vi "Auto_Routine_StraightTwoPiece.vi"(8 "error in (no error)":errorcluster) -> (0 "error out":errorcluster)   [LabVIEW 2023]
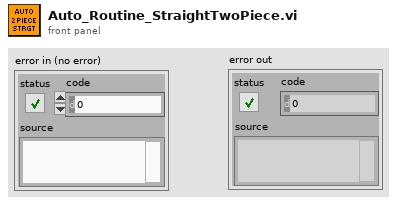
[diagram p1: front panel]
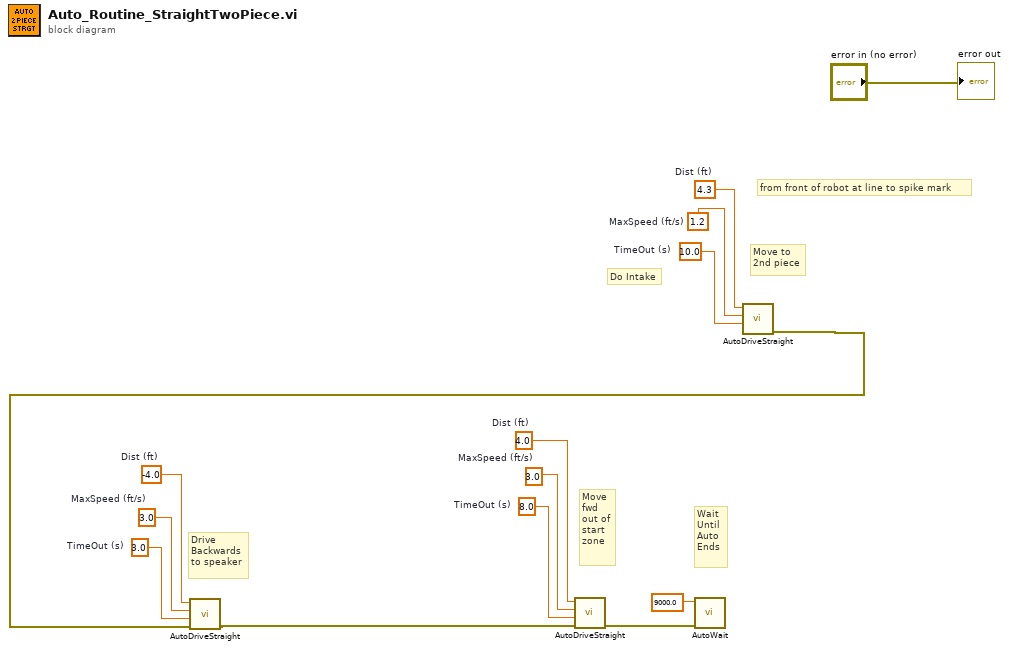
[diagram p0: block diagram]
diagram:
  w13 = 8.0  # TimeOut (s)
  w12 = 3.0  # MaxSpeed (ft/s)
  w11 = 4.0  # Dist (ft)
  w10 = 3.0  # TimeOut (s)
  w9 = 3.0  # MaxSpeed (ft/s)
  w8 = -4.0  # Dist (ft)
  w6 = 10.0  # TimeOut (s)
  w5 = 1.2  # MaxSpeed (ft/s)
  w4 = 4.3  # Dist (ft)
  # "Wait\nUntil\nAuto \nEnds"
  # "Move\nfwd\nout of\nstart\nzone"
  # "Drive\nBackwards\nto speaker"
  # "Do Intake"
  # "Move to \n2nd piece"
  # "from front of robot at line to spike mark"
  n1 = call "AutoDriveStraight.vi"("TimeOut (s)"=w6, "MaxSpeed (ft/s)"=w5, "Dist (ft)"=w4) -> ("error out"=w2:errorcluster)  [unwired: 8 in]
  n2 = call "AutoDriveStraight.vi"("error in (no error)"=w2, "TimeOut (s)"=w10, "MaxSpeed (ft/s)"=w9, "Dist (ft)"=w8) -> ("error out"=w1:errorcluster)  [unwired: 7 in]
  n3 = call "AutoDriveStraight.vi"("error in (no error)"=w1, "TimeOut (s)"=w13, "MaxSpeed (ft/s)"=w12, "Dist (ft)"=w11) -> ("error out"=w14:errorcluster)  [unwired: 7 in]
  n4 = call "AutoWait.vi"("error in (no error)"=w14, "TimeOut (s)"=9000.0) -> ()  [unwired: 9 in, 1 out]
  "error out" <- "error in (no error)"
